vi "N-565 Stage Engine.vi"(0 "Unique Notifier Name":string, 11 "COM Port":string[](array[string])) -> ()   [LabVIEW 2016]
uses:
  Stages Controls/Stage Focus Control.ctl
  Stages Controls/Stage Status.ctl
  Stages Controls/Stage Notifier Element.ctl
  Stages Controls/Stage Actions.ctl
panel:
  in  "ReInitialize":bool
  in  "Abort":bool
  in  "Velocity":dbl(ring)=2.0 items=["SUPER SLOW"=0.0010000000474974513, "SLOW"=1.0, "MEDIUM"=2.0, "FAST"=3.0]
  out "Status":T1
  in  "QUIT":bool
  in  "Focus Control":T2
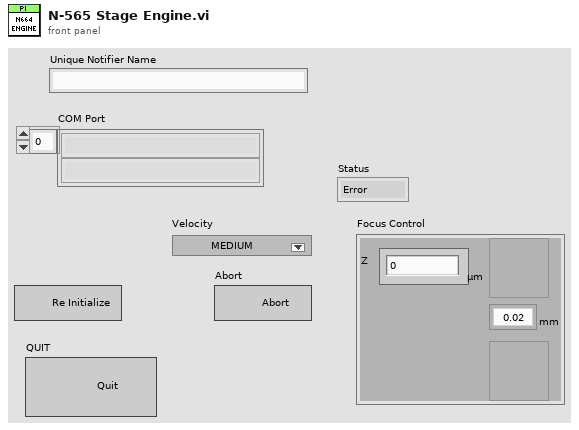
[diagram p1: front panel]
types:
  T1 = typedef "Stage Status.ctl" = enum16{"Error", "Abort", "Busy", "On Target"}
  T2 = typedef "Stage Focus Control.ctl" = cluster{"Focus Step (um)":enum16{"0.02", "0.05", "0.1", "0.5", "1", "2", "5", "10", "20"}, "Focus Up":bool, "Focus Down":bool, "Z ":dbl}
  T3 = typedef "Stage Actions.ctl" = enum16{"Get Position", "MVR", "MOVE", "HALT", "ONTARGET", "ERROR", "REFERENCE", "INIT", "VELOCITY", "STATUS", "EXIT", "HOME", "ZEROPOS", "NANOPOS", "ANALOG", "QUIT"}
  T4 = typedef "Stage Notifier Element.ctl" = cluster{"Action":T3, "Axis":bool[], "Setpoint":dbl[], "Velocity":dbl, "Cmd Recvd?":bool, "Position":dbl[], "Status":T1, "Misc":variant}
  T5 = cluster{"Focus Step (um)":bool, "Focus Up":bool, "Focus Down":bool, "Z ":bool}
  T6 = enum16{"0.02", "0.05", "0.1", "0.5", "1", "2", "5", "10", "20"}
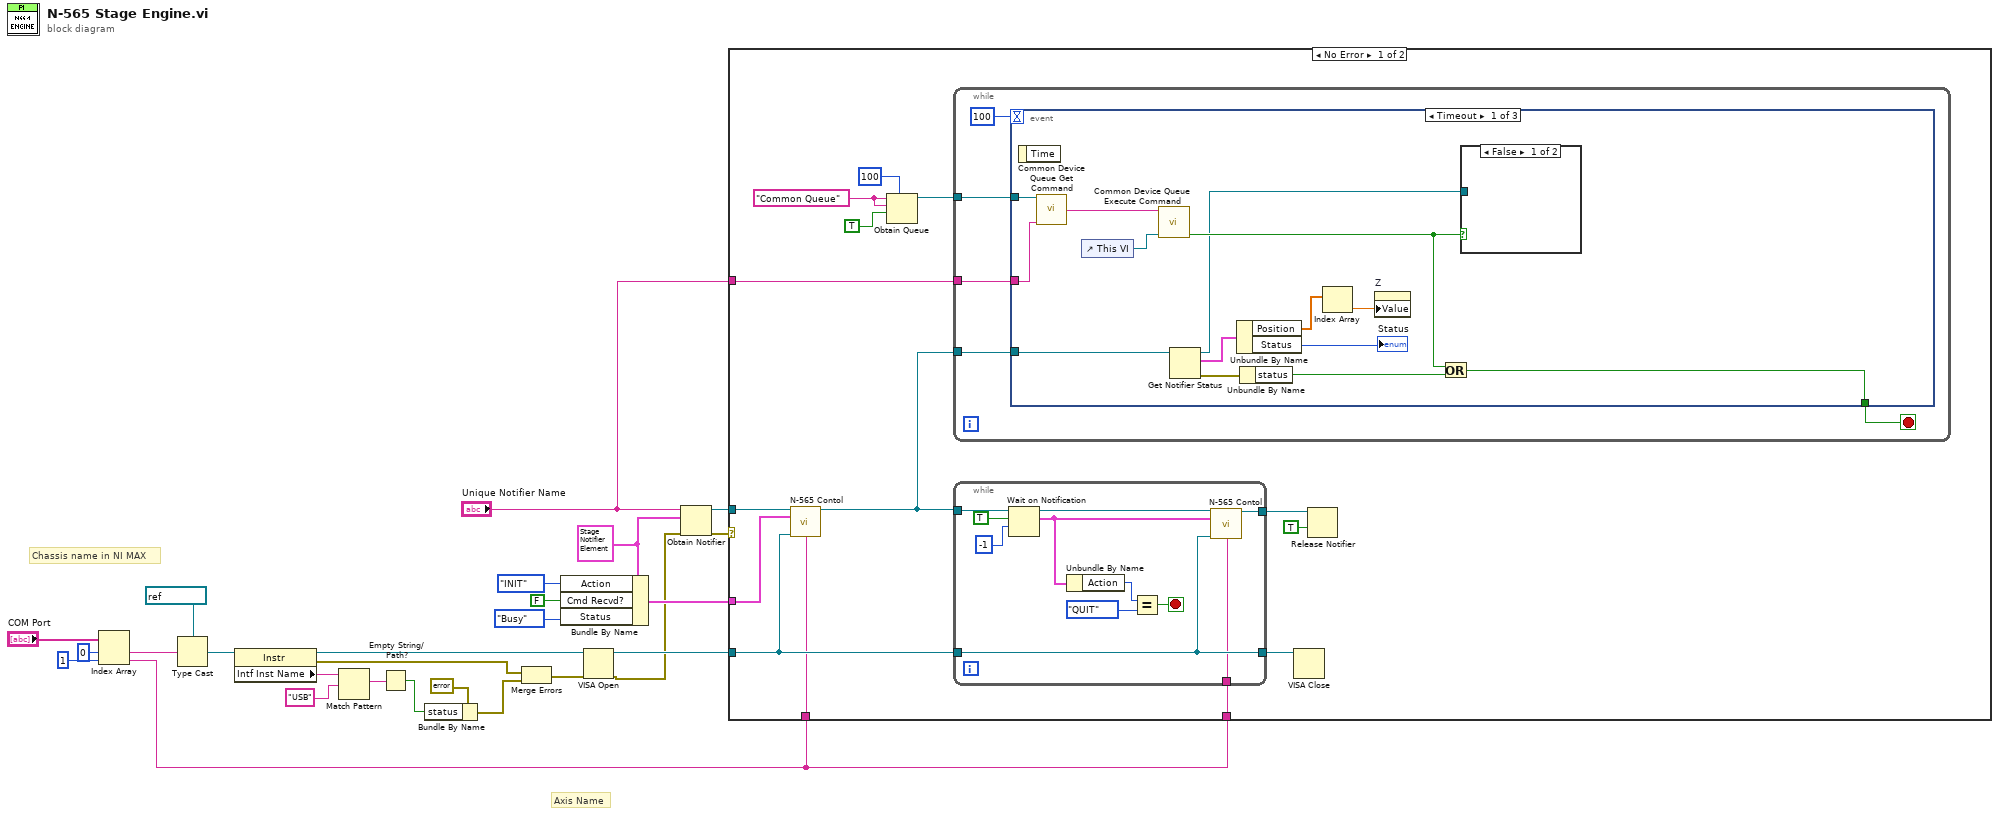
[diagram p0: block diagram]
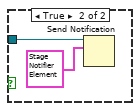
[diagram p2: hidden frame]
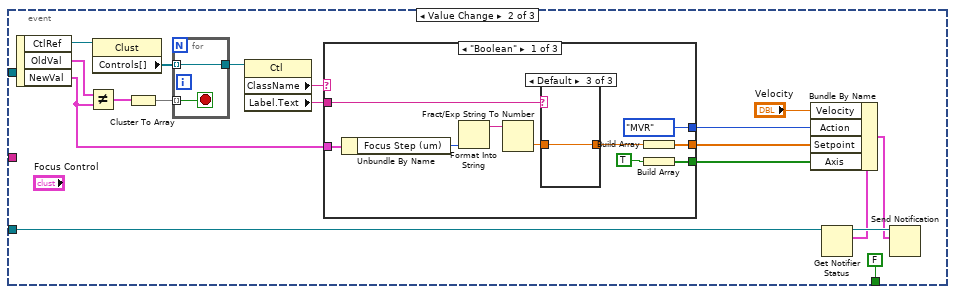
[diagram p3: hidden frame]
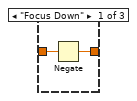
[diagram p4: hidden frame]
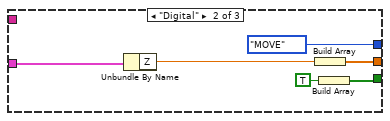
[diagram p6: hidden frame]
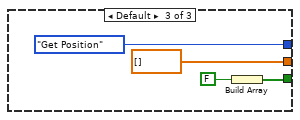
[diagram p7: hidden frame]
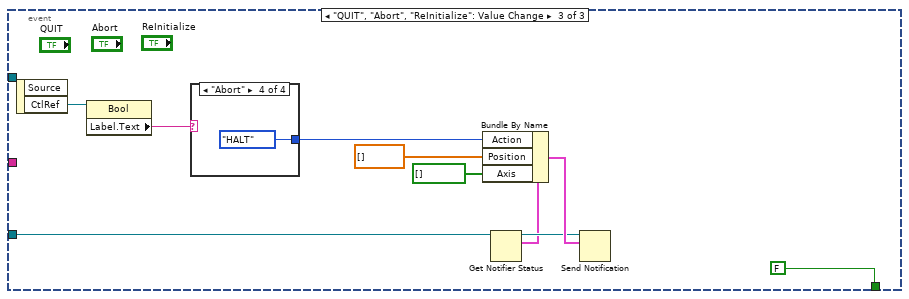
[diagram p8: hidden frame]
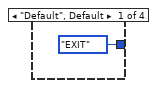
[diagram p9: hidden frame]
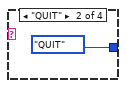
[diagram p10: hidden frame]
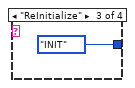
[diagram p11: hidden frame]
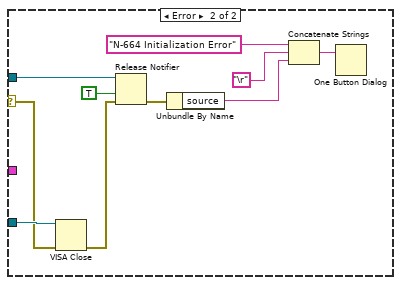
[diagram p12: hidden frame]
diagram:
  w12 = T4 {"Action"=enum."Get Position", "Axis"=[], "Setpoint"=[], "Velocity"=0.5, "Cmd Recvd?"=FALSE, "Position"=[], "Status"=enum."Abort", "Misc"=variant} ("Stage Status")
  # "Axis Name"
  # "Chassis name in NI MAX"
  n1 = Index Array(array="COM Port", index #1=0 ("index"), index #2=1 ("index")) -> (element #1=w20:string, element #2=w5:string)
  n2 = Type Cast(type=refnum<visa-resource-name> "COM6" ("reference out"), x=w20) -> (*(type *) &x=w18:refnum<visa-resource-name>)
  n3 = property class="Instr"(reference=w18) -> (reference out=w4:refnum<visa-resource-name>, error out=w22:errorcluster, "Intf Inst Name"=w24:string)  [unwired: 1 in]
  n4 = Match Pattern(string=w24, regular expression="USB") -> (match substring=w26:string)  [unwired: 1 in, 3 out]
  n5 = Empty String/Path?(string/path=w26) -> (empty?=w23:bool)
  n6 = Bundle By Name(cluster=errorcluster {"status"=FALSE, "code"=0, "source"=""} ("Error"), "status"=w23) -> (w16:errorcluster)
  n7 = Merge Errors(w22, w16) -> (w2:errorcluster)
  n8 = Bundle By Name(cluster=w12, "Action"=Stage_Actions."INIT", "Cmd Recvd?"=FALSE, "Status"=Stage_Status."Busy") -> (w9:T4)
  n9 = VISA Open(error in (no error)=w2, VISA resource name=w4) -> (VISA resource name=w3:refnum<visa-resource-name>, error out=w1:errorcluster)  [unwired: 3 in]
  n10 = Obtain Notifier(name (unnamed)="Unique Notifier Name", notification data type=w12, error in (no error)=w1) -> (notifier out=w11:refnum<notifier>, error out=w10:errorcluster)  [unwired: 1 in, 1 out]
  n11 = case shown="No Error" w10 {
    selector: w10 -> [_ w131]
    tunnel: w3 -> [w35 w132]
    tunnel: w11 -> [w39 w133]
    tunnel: w9 -> [w38 _]
    tunnel: "Unique Notifier Name" -> [w29 _]
    tunnel: w5 -> [w28 _]
    tunnel: w5 -> [w27 _]
    frame No Error {
      w33 = "Common Queue" ("Unique Notifier Name")
      n12 = call "N-565 Contol.vi"("N-664 Notifier"=w39, "Stage Action"=w38, "VISA In"=w35, "Axis Name"=w27) -> ("N-664 Notifier (Dup)"=w37:refnum<notifier>)  [unwired: 11 in]
      n13 = Obtain Queue(max queue size (-1, unlimited)=100, name (unnamed)=w33, element data type=w33, create if not found? (T)=TRUE) -> (queue out=w30:refnum<queue>)  [unwired: 1 in, 2 out]
      n14 = while {
        tunnel: w37 -> [w54]
        tunnel: w30 -> [w53]
        tunnel: w29 -> [w52]
        stop <- w55 stop-if-true
        n15 = event shown="[0] Timeout" {
          selector: _ -> [_ _ _]
          dyn-events: _ -> [_ _ _]
          timeout: 100 -> [_ _ _]
          tunnel: [w60 FALSE ("status") FALSE ("status")] -> w55
          tunnel: w54 -> [w69 w78 w122]
          tunnel: w53 -> [w62 _ _]
          tunnel: w52 -> [w57 _ _]
          event Timeout {
            n16 = event-data() -> ()  [unwired: 1 in, 1 out]
            n17 = call "Common Device Queue Get Command.vi"("Common Queue"=w62, "Notifier Name"=w57) -> ("Command"=w63:string)  [unwired: 12 in, 1 out]
            n18 = control-ref of="This VI"() -> (w64:refnum<vi>)
            n19 = call "Common Device Queue Execute Command.vi"("Common Command"=w63, "VI Refnum"=w64) -> ("Quit?"=w59:bool)  [unwired: 12 in, 1 out]
            n20 = Get Notifier Status(notifier=w69) -> (notifier out=w58:refnum<notifier>, current notification=w68:T4, error out=w66:errorcluster)  [unwired: 1 in, 2 out]
            n21 = Unbundle By Name(w68) -> ("Position"=w67:dbl[], "Status"=→"Status":T1)
            n22 = Unbundle By Name(w66) -> ("status"=w61:bool)
            n23 = Index Array(array=w67) -> (element=w70:dbl)  [unwired: 1 in]
            n24 = property on="Z" class="DigNum (strict)"("Value"=w70) -> ()  [unwired: 2 in, 2 out]
            n25 = Or(x=w59, y=w61) -> (x .or. y?=w60:bool)
            n26 = case shown="False" w59 {
              tunnel: w58 -> [_ w72]
              frame False {
              }
              frame True {
                n27 = Send Notification(notification=T4 {"Action"=enum."QUIT", "Axis"=[], "Setpoint"=[], "Velocity"=0.5, "Cmd Recvd?"=FALSE, "Position"=[], "Status"=enum."Error", "Misc"=variant} ("Stage Status"), notifier=w72) -> ()  [unwired: 1 in, 2 out]
              }
            }
          }
          event Value Change {
            n28 = event-data() -> ("CtlRef"=w89:refnum<vi>, "OldVal"=w90:T2, "NewVal"=w83:T2)  [unwired: 1 in]
            n29 = Not Equal?(x=w90, y=w83) -> (x != y?=w88:T5)
            n30 = property class="Clust"(reference=w89) -> ("Controls[]"=w86:refnum<vi>[])  [unwired: 1 in, 2 out]
            n31 = Cluster To Array(cluster=w88) -> (array=w87:bool[])
            n32 = for {
              tunnel: w87 -> [w116] mode=indexing
              tunnel: [w115] -> w85
              tunnel: w86 -> [w115] mode=indexing
              stop <- w116 stop-if-true
            }
            n33 = property class="Ctl"(reference=w85) -> ("ClassName"=w84:string, "Label.Text"=w82:string)  [unwired: 1 in, 2 out]
            n34 = case shown="\"Boolean\"" w84 {
              tunnel: w83 -> [w98 w110 _]
              tunnel: w82 -> [w99 _ _]
              tunnel: [w93 w108 dbl[] []] -> w81
              tunnel: [w92 w107 w113] -> w80
              tunnel: [Stage_Actions."MVR" ("Action") Stage_Actions."MOVE" ("Action") Stage_Actions."Get Position" ("Action")] -> w77
              frame "Boolean" {
                n35 = Unbundle By Name(w98) -> ("Focus Step (um)"=w96:T6)
                n36 = Format Into String(w96) -> (resulting string=w97:string)  [unwired: 3 in, 1 out]
                n37 = Fract/Exp String To Number(string=w97) -> (number=w95:dbl)  [unwired: 3 in, 1 out]
                n38 = case shown="Default" w99 {
                  tunnel: w95 -> [w102 w103 w104]
                  tunnel: [w101 w103 w104] -> w94
                  frame "Focus Down" {
                    n39 = Negate(x=w102) -> (-x=w101:dbl)
                  }
                  frame "Focus Up" {
                  }
                  frame Default {
                  }
                }
                n40 = Build Array(w94) -> (w93:dbl[])
                n41 = Build Array(TRUE) -> (w92:bool[])
              }
              frame "Digital" {
                n42 = Unbundle By Name(w110) -> ("Z"=w109:dbl)
                n43 = Build Array(w109) -> (w108:dbl[])
                n44 = Build Array(TRUE) -> (w107:bool[])
              }
              frame Default {
                n45 = Build Array(FALSE) -> (w113:bool[])
              }
            }
            n46 = Get Notifier Status(notifier=w78) -> (notifier out=w76:refnum<notifier>, current notification=w75:T4)  [unwired: 1 in, 3 out]
            n47 = Bundle By Name(cluster=w75, "Velocity"="Velocity", "Action"=w77, "Setpoint"=w81, "Axis"=w80) -> (w74:T4)
            n48 = Send Notification(notification=w74, notifier=w76) -> ()  [unwired: 1 in, 2 out]
          }
          event "QUIT", "Abort", "ReInitialize": Value Change {
            n49 = event-data() -> ("CtlRef"=w119:refnum<vi>)  [unwired: 1 in, 1 out]
            n50 = property class="Bool"(reference=w119) -> ("Label.Text"=w118:string)  [unwired: 1 in, 2 out]
            n51 = case shown="\"Abort\"" w118 {
              tunnel: [Stage_Actions."EXIT" ("Action") Stage_Actions."QUIT" ("Action") Stage_Actions."INIT" ("Action") Stage_Actions."HALT" ("Action")] -> w117
              frame "Default", Default {
              }
              frame "QUIT" {
              }
              frame "ReInitialize" {
              }
              frame "Abort" {
              }
            }
            n52 = Get Notifier Status(notifier=w122) -> (notifier out=w121:refnum<notifier>, current notification=w120:T4)  [unwired: 1 in, 3 out]
            n53 = Bundle By Name(cluster=w120, "Action"=w117, "Position"=dbl[] [], "Axis"=bool[] []) -> (w123:T4)
            n54 = Send Notification(notification=w123, notifier=w121) -> ()  [unwired: 1 in, 2 out]
          }
        }
      }
      n55 = while {
        tunnel: w37 -> [w49]
        tunnel: [w45] -> w36
        tunnel: w35 -> [w44]
        tunnel: [w44] -> w34
        tunnel: w28 -> [w41]
        stop <- w51 stop-if-true
        n56 = Wait on Notification(notifier=w49, ignore previous (F)=TRUE, timeout in ms (-1)=-1) -> (notifier out=w46:refnum<notifier>, notification=w43:T4)  [unwired: 1 in, 2 out]
        n57 = Unbundle By Name(w43) -> ("Action"=w42:T3)
        n58 = Equal?(x=w42, y=Stage_Actions."QUIT") -> (x = y?=w51:bool)
        n59 = call "N-565 Contol.vi"("N-664 Notifier"=w46, "Stage Action"=w43, "VISA In"=w44, "Axis Name"=w41) -> ("N-664 Notifier (Dup)"=w45:refnum<notifier>)  [unwired: 11 in]
      }
      n60 = VISA Close(VISA resource name=w34) -> ()  [unwired: 1 in, 1 out]
      n61 = Release Notifier(notifier=w36, force destroy? (F)=TRUE) -> ()  [unwired: 1 in, 3 out]
    }
    frame Error {
      n62 = VISA Close(VISA resource name=w132, error in (no error)=w131) -> (error out=w134:errorcluster)
      n63 = Release Notifier(notifier=w133, force destroy? (F)=TRUE, error in (no error)=w134) -> (error out=w139:errorcluster)  [unwired: 2 out]
      n64 = Unbundle By Name(w139) -> ("source"=w136:string)
      n65 = Concatenate Strings("N-664 Initialization Error", "\r", w136) -> (w135:string)
      n66 = One Button Dialog(message=w135) -> ()  [unwired: 1 in, 1 out]
    }
  }
